vi "rep_cap_find_name.vi"(5 "Operation":T1(ring)=enum."Get Cmd Value", 6 "error creation enabled (T)":bool=TRUE, 7 "RepCapNames in":string[](array[string]), 8 "error in":errorcluster, 10 "RepCapNameID for error msg (\"\")":string, 11 "RepCapName to search":string) -> (0 "error out":errorcluster, 3 "Index out":i32)   [LabVIEW 2014, in "rszvl_rsidr_core.lvlib"]
uses:
  rszvl_rsidr_core.lvlib
  type_Error_Codes.ctl
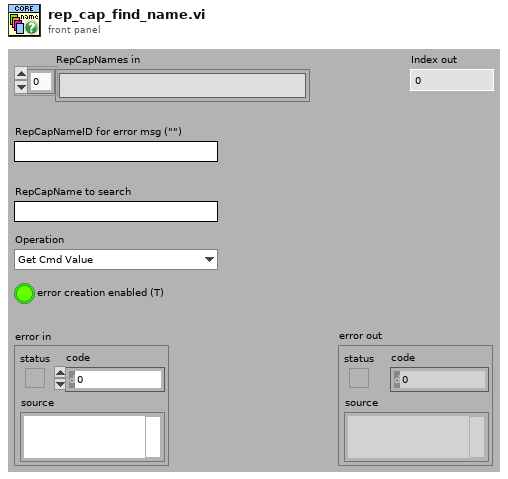
[diagram p1: front panel]
types:
  T1 = enum16{"Initialize", "Get Cmd Value", "Reset Rep Cap", "Add Rep Cap", "Remove Rep Cap", "Get Rep Cap ID range", "Get Count", "Clear", "Find Name from NameID", "Get First NameID"}
  T2 = typedef "rszvl_rsidr_core.lvlib/type_Error_Codes.ctl" = enum16{"No_error", "VISA_err_ResourceNotFound", "VISA_err_Timeout", "VISA_warn_MoreDataAvailable", "RS_err_MissingCallback", "RS_err_InvalidAttribute", "RS_err_InvalidValue", "RS_err_UnknownResource", "RS_err_AlreadyInitialized", "RS_err_InstrumentStatus", "RS_err_BadRepCapName", "RS_err_TypesMismatch", "RS_err_ValueNotSupported", "RS_err_InvalidRngTable", "RS_err_IDqueryFail", "RS_err_UnexpResponse", "VISA_warn_ConfigNotLoaded", "RS_err_AttributeNotReadable", "RS_err_AttributeNotWritable", "RS_err_InstrumentType", "RS_err_InstrumentOption", "VISA_err_InvalidSize", "RS_err_ReliabilityIndicator", "VISA_warn_UnknownStatus", "VISA_warn_TermCharRead", "VISA_err_IO_error"}
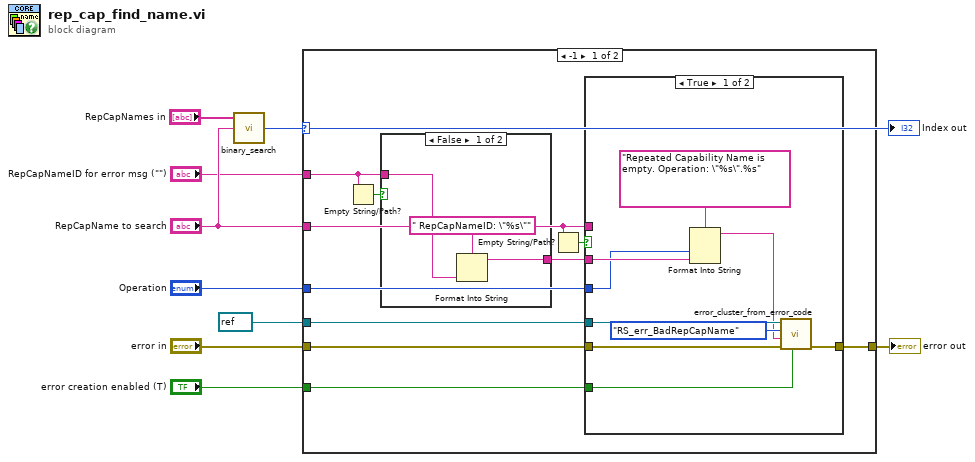
[diagram p0: block diagram]
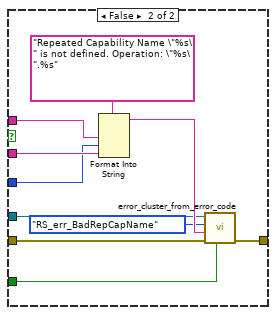
[diagram p3: hidden frame]
diagram:
  n1 = call "binary_search.vi"("String to search"="RepCapName to search", "Strings in"="RepCapNames in") -> ("Index out"=w9:i32)  [unwired: 3 in]
  "Index out" <- w9
  n2 = case shown="-1" w9 {
    tunnel: [w18 w42] -> w4
    tunnel: "error in" -> [w19 w42]
    tunnel: "RepCapName to search" -> [w16 _]
    tunnel: "RepCapNameID for error msg (\"\")" -> [w14 _]
    tunnel: "Operation" -> [w12 _]
    tunnel: refnum<visa-resource-name> refnum ("VISA resource name") -> [w11 _]
    tunnel: "error creation enabled (T)" -> [w10 _]
    frame -1 {
      n3 = Empty String/Path?(string/path=w14) -> (empty?=w15:bool)
      n4 = case shown="False" w15 {
        tunnel: w14 -> [w21 _]
        tunnel: [w20 _] -> w13
        frame False {
          n5 = Format Into String(format string=" RepCapNameID: \"%s\"", w21) -> (resulting string=w20:string)  [unwired: 2 in, 1 out]
        }
        frame True {
        }
      }
      n6 = Empty String/Path?(string/path=w16) -> (empty?=w17:bool)
      n7 = case shown="True" w17 {
        tunnel: w19 -> [w31 w41]
        tunnel: [w30 w40] -> w18
        tunnel: w16 -> [_ w37]
        tunnel: w13 -> [w28 w39]
        tunnel: w12 -> [w27 w38]
        tunnel: w11 -> [w25 w34]
        tunnel: w10 -> [w23 w32]
        frame True {
          n8 = Format Into String(format string="Repeated Capability Name is empty. Operation: \"%s\".%s", w27, w28) -> (resulting string=w24:string)  [unwired: 2 in, 1 out]
          n9 = call "error_cluster_from_error_code.vi"("error creation enabled (T)"=w23, "error in"=w31, "error message (\"\")"=w24, "Error Enum in"=type_Error_Codes."RS_err_BadRepCapName", "VISA resource name"=w25) -> ("error out"=w30:errorcluster)  [unwired: 5 in, 1 out]
        }
        frame False {
          n10 = Format Into String(format string="Repeated Capability Name \"%s\" is not defined. Operation: \"%s\".%s", w37, w38, w39) -> (resulting string=w35:string)  [unwired: 2 in, 1 out]
          n11 = call "error_cluster_from_error_code.vi"("error creation enabled (T)"=w32, "error in"=w41, "error message (\"\")"=w35, "Error Enum in"=type_Error_Codes."RS_err_BadRepCapName", "VISA resource name"=w34) -> ("error out"=w40:errorcluster)  [unwired: 5 in, 1 out]
        }
      }
    }
    frame Default {
    }
  }
  "error out" <- w4
